vi "Triggered Tasks-Stop only.vi"() -> (0 "error out":errorcluster)   [LabVIEW 2020]
uses:
  Globals/gl_Triggering globals.vi
  Pockels/Globals/gl_Pockels control globals.vi
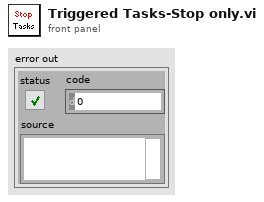
[diagram p1: front panel]
types:
  T1 = typedef "Triggered tasks cluster.ctl" = cluster{"DO task-Encoder trigger":refnum<k21>, "AO Task-Pockels modulation":refnum<k21>, "Counter Clock Task":refnum<k21>}
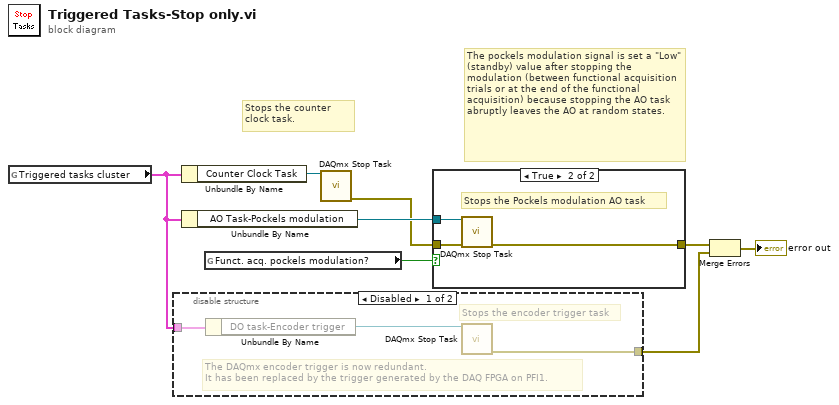
[diagram p0: block diagram]
diagram:
  # "The pockels modulation signal is set a \"Low\" (standby) value after stopping the modulation (between functional acquisition trials or at the end of the functional acquisition) because stopping the AO task abruptly leaves the AO at random states."
  # "Stops the counter clock task."
  n1 = global read "gl_Triggering globals.vi" "Triggered tasks cluster"() -> (w4:T1)
  n2 = disable-structure shown="Disabled" {
    disable-tunnel: w4 -> [w10 _]
    disable-tunnel: [w9 _] -> w2
    frame Disabled {
      # "The DAQmx encoder trigger is now redundant.\nIt has been replaced by the trigger generated by the DAQ FPGA on PFI1."
      # "Stops the encoder trigger task"
      n3 = Unbundle By Name(w10) -> ("DO task-Encoder trigger"=w11:refnum<k21>)
      n4 = call <vilib>:"DAQmx Stop Task.vi"("task/channels in"=w11) -> ("error out"=w9:errorcluster)  [unwired: 13 in, 1 out]
    }
    frame Enabled {
    }
  }
  n5 = Unbundle By Name(w4) -> ("Counter Clock Task"=w7:refnum<k21>)
  n6 = Unbundle By Name(w4) -> ("AO Task-Pockels modulation"=w5:refnum<k21>)
  n7 = global read "gl_Pockels control globals.vi" "Funct. acq. pockels modulation?"() -> (w6:bool)
  n8 = call <vilib>:"DAQmx Stop Task.vi"("task/channels in"=w7) -> ("error out"=w1:errorcluster)  [unwired: 13 in, 1 out]
  n9 = case shown="True" w6 {
    tunnel: [w12 w13] -> w8
    tunnel: w5 -> [_ w15]
    tunnel: w1 -> [w12 w14]
    frame False {
    }
    frame True {
      # "Stops the Pockels modulation AO task"
      n10 = call <vilib>:"DAQmx Stop Task.vi"("task/channels in"=w15, "error in"=w14) -> ("error out"=w13:errorcluster)  [unwired: 12 in, 1 out]
    }
  }
  n11 = Merge Errors(w8, w2) -> (→"error out":errorcluster)
